vi "Tosca-Initialize Stimulus Generation.vi"(0 "Tosca":refnum<class "Parameters.lvclass">, 1 "StimCon in":T1, 11 "error in (no error)":errorcluster, 12 "SG Runtime":T7) -> (3 "StimCon out":T1, 4 "Tosca out":refnum<class "Parameters.lvclass">, 8 "AODO":T4[](array[typedef]), 15 "error out":errorcluster)   [LabVIEW 2020]
uses:
  Typedefs/Tosca-SG Runtime Params.ctl
  Typedefs/Tosca-AO Runtime.ctl
  Typedefs/Tosca-DO Runtime.ctl
  Imaging VIs/Tosca-Imaging Mode.ctl
  Classes/Parameters/Parameters.lvclass
  Typedefs/Tosca-State AODO.ctl
  epl-vi-lib/Signal Synthesis VIs/4th Generation/Classes/SignalManager/SignalManager.lvclass
  Typedefs/Tosca-SCL Element.ctl
  Typedefs/Tosca-Schedule Mode.ctl
  Typedefs/Tosca-Event Type.ctl
  Classes/Parameters/Parameters.lvclass/Parameters.ctl
  Classes/State/State.lvclass/State.ctl
  epl-vi-lib/Signal Synthesis VIs/4th Generation/Classes/SignalManager/SignalManager.lvclass/SignalManager.ctl
  Classes/State/Read Name.vi
  Classes/State/Read SigMan.vi
  epl-vi-lib/Signal Synthesis VIs/4th Generation/Classes/SignalManager/Read Interval (ms).vi
  Classes/Parameters/Read First state.vi
  Classes/Parameters/Read Flowchart.vi
  Classes/Parameters/Read DAQ.vi
  Classes/State/State.lvclass
  epl-vi-lib/PXI DAQ VIs/AODO/Typedefs/AODO-Action.ctl
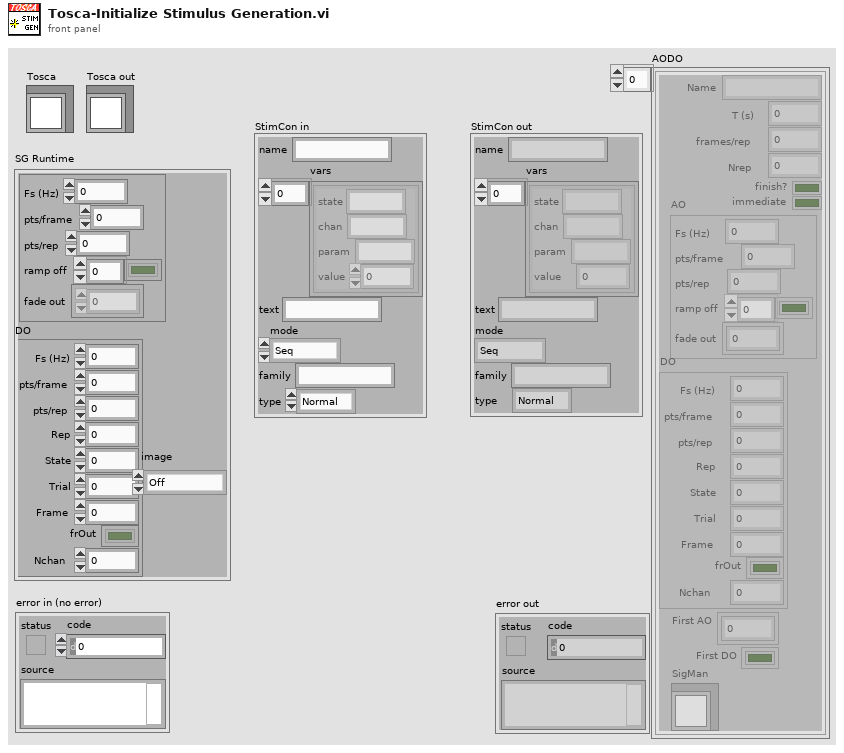
[diagram p1: front panel]
types:
  T1 = typedef "Tosca-SCL Element.ctl" = cluster{"name":string, "vars":cluster{"state":string, "chan":string, "param":string, "value":dbl}[], "text":string, "mode":T2, "family":string, "type":T3}
  T2 = typedef "Tosca-Schedule Mode.ctl" = enum16{"Seq", "CS+/CS-", "Adapt"}
  T3 = typedef "Tosca-Event Type.ctl" = enum16{"Normal", "CS+", "CS-"}
  T4 = typedef "Tosca-State AODO.ctl" = cluster{"Name":string, "T (s)":dbl, "First AO":dbl[][], "frames/rep":i32, "finish?":bool, "Nrep":i32, "AO":T5, "DO":T6, "immediate":bool, "First DO":bool[][], "SigMan":refnum<class "SignalManager.lvclass">}
  T5 = typedef "Tosca-AO Runtime.ctl" = cluster{"Fs (Hz)":dbl, "pts/frame":i32, "pts/rep":i32, "ramp off":bool[], "fade out":dbl[][]}
  T6 = typedef "Tosca-DO Runtime.ctl" = cluster{"Fs (Hz)":dbl, "pts/frame":i32, "pts/rep":i32, "Rep":i32, "State":i32, "Trial":i32, "Frame":i32, "frOut":bool[], "Nchan":i32}
  T7 = typedef "Tosca-SG Runtime Params.ctl" = cluster{"AO":T5, "DO":T6, "image":T8}
  T8 = typedef "Tosca-Imaging Mode.ctl" = enum16{"Off", "Widefield", "Two-photon"}
  T9 = typedef "Parameters.lvclass/DAQ.ctl" = cluster{"AO Fs (Hz)":dbl, "DO Fs (Hz)":dbl, "Poll Rate (Hz)":dbl, "Baseline (s)":dbl}
  T10 = typedef "AODO-Action.ctl" = enum16{"Configure", "Initialize", "Start", "Write", "Clean up", "Init & Start", "Config & Test", "Position", "Set AO Gains", "Zero"}
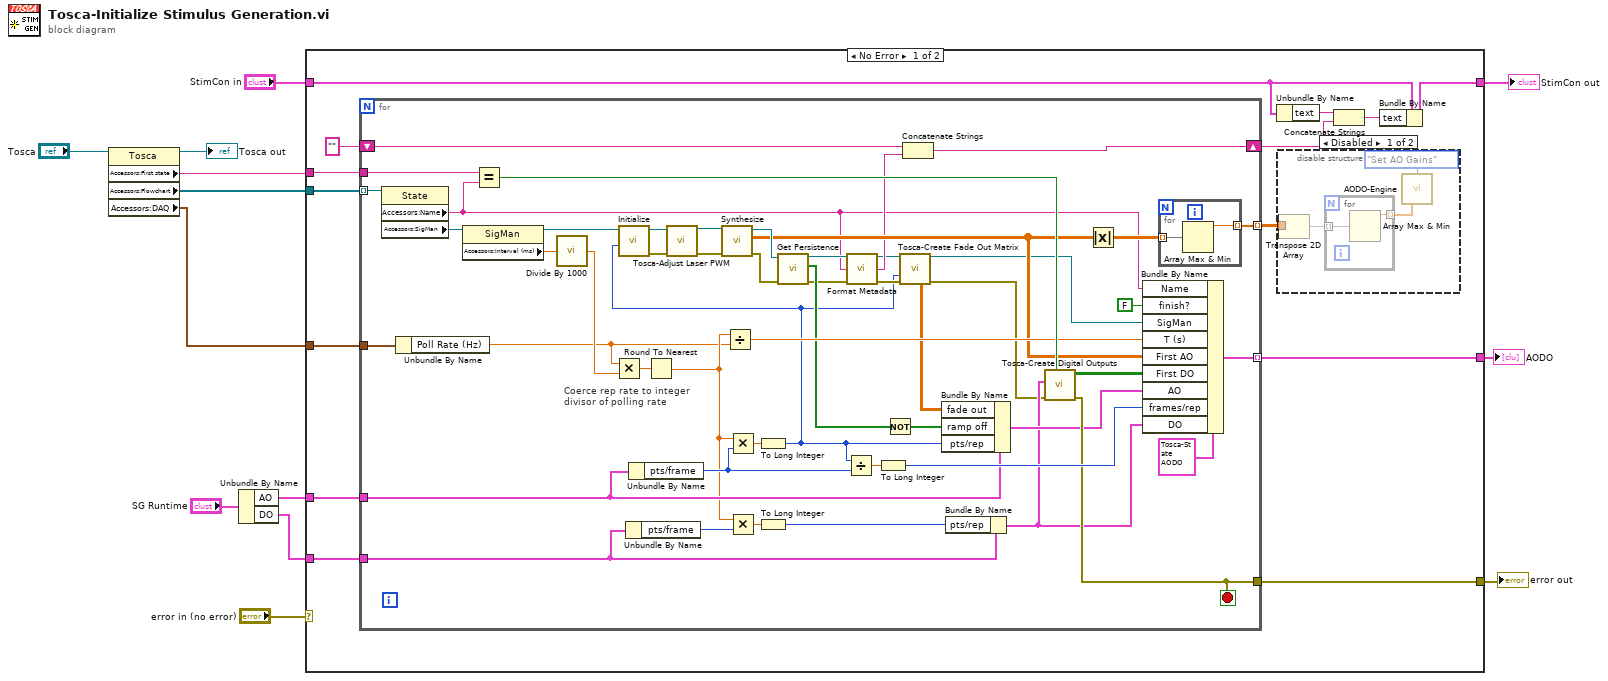
[diagram p0: block diagram]
diagram:
  n1 = property class="Tosca"(reference="Tosca") -> (reference out=→"Tosca out":refnum<class "Parameters.lvclass">, "Accessors:First state"=w7:string, "Accessors:Flowchart"=w8:refnum<class "State.lvclass">[], "Accessors:DAQ"=w4:T9)  [unwired: 1 in, 1 out]
  n2 = Unbundle By Name("SG Runtime") -> ("AO"=w11:T5, "DO"=w10:T6)
  n3 = case shown="No Error" "error in (no error)" {
    selector: "error in (no error)" -> [_ w88]
    tunnel: [w25 w88] -> w12
    tunnel: [w22 _] -> w3
    tunnel: w11 -> [w27 _]
    tunnel: w10 -> [w26 _]
    tunnel: w8 -> [w24 _]
    tunnel: w7 -> [w23 _]
    tunnel: w4 -> [w21 _]
    tunnel: [w18 w87] -> w2
    tunnel: "StimCon in" -> [w17 w87]
    frame No Error {
      n4 = for {
        tunnel: w27 -> [w73]
        tunnel: w26 -> [w65]
        tunnel: [w69] -> w25
        tunnel: w24 -> [w61] mode=indexing
        tunnel: w23 -> [w57]
        tunnel: [w55] -> w22 mode=indexing
        tunnel: w21 -> [w54]
        tunnel: [w49] -> w20 mode=indexing
        shift-right: [w36] -> w15
        shift-left: "" -> [w39]
        stop <- w69 stop-if-true
        # "Coerce rep rate to integer divisor of polling rate"
        n5 = property class="State"(reference=w61) -> ("Accessors:Name"=w34:string, "Accessors:SigMan"=w58:refnum<class "SignalManager.lvclass">)  [unwired: 1 in, 2 out]
        n6 = Unbundle By Name(w54) -> ("Poll Rate (Hz)"=w53:dbl)
        n7 = property class="SigMan"(reference=w58) -> (reference out=w56:refnum<class "SignalManager.lvclass">, "Accessors:Interval (ms)"=w60:dbl)  [unwired: 1 in, 1 out]
        n8 = Equal?(x=w57, y=w34) -> (x = y?=w70:bool)
        n9 = call "Divide By 1000.vi"("X"=w60) -> ("X/1000"=w59:dbl)
        n10 = Multiply(x=w53, y=w59) -> (x*y=w78:dbl)
        n11 = Unbundle By Name(w65) -> ("pts/frame"=w62:i32)
        n12 = Unbundle By Name(w73) -> ("pts/frame"=w66:i32)
        n13 = Round To Nearest(number=w78) -> (nearest integer value=w63:dbl)
        n14 = Divide(x=w63, y=w53) -> (x/y=w64:dbl)
        n15 = Multiply(x=w63, y=w66) -> (x*y=w77:dbl)
        n16 = Multiply(x=w63, y=w62) -> (x*y=w74:dbl)
        n17 = To Long Integer(number=w77) -> (32bit integer=w29:i32)
        n18 = call "Initialize.vi"("Npts"=w29, "SigMan in"=w56) -> ("error out"=w46:errorcluster, "SigMan out"=w48:refnum<class "SignalManager.lvclass">)  [unwired: 8 in]
        n19 = call "Tosca-Adjust Laser PWM.vi"("SigMan in"=w48, "error in (no error)"=w46) -> ("SigMan out"=w47:refnum<class "SignalManager.lvclass">, "error out"=w45:errorcluster)  [unwired: 12 in]
        n20 = call "Synthesize.vi"("error in (no error)"=w45, "SigMan in"=w47) -> ("error out"=w44:errorcluster, "Array"=w40:dbl[][], "SigMan out"=w43:refnum<class "SignalManager.lvclass">)  [unwired: 7 in]
        n21 = To Long Integer(number=w74) -> (32bit integer=w72:i32)
        n22 = call "Get Persistence.vi"("error in (no error)"=w44, "SigMan in"=w43) -> ("error out"=w38:errorcluster, "persist"=w42:bool[], "SigMan out"=w37:refnum<class "SignalManager.lvclass">)  [unwired: 7 in]
        n23 = Divide(x=w29, y=w66) -> (x/y=w76:dbl)
        n24 = call "Format Metadata.vi"("SigMan in"=w37, "Prefix"=w34, "error in (no error)"=w38) -> ("SigMan out"=w32:refnum<class "SignalManager.lvclass">, "String"=w35:string, "error out"=w33:errorcluster)  [unwired: 10 in]
        n25 = To Long Integer(number=w76) -> (32bit integer=w75:i32)
        n26 = Not(x=w42) -> (.not. x?=w41:bool[])
        n27 = call "Tosca-Create Fade Out Matrix.vi"("SignalManager in"=w32, "npts"=w29, "error in (no error)"=w33) -> ("SignalManager out"=w31:refnum<class "SignalManager.lvclass">, "fade out"=w28:dbl[][], "error out"=w30:errorcluster)  [unwired: 10 in]
        n28 = Concatenate Strings(w39, w35) -> (w36:string)
        n29 = Bundle By Name(cluster=w73, "fade out"=w28, "ramp off"=w41, "pts/rep"=w29) -> (w68:T5)
        n30 = Bundle By Name(cluster=w65, "pts/rep"=w72) -> (w67:T6)
        n31 = call "Tosca-Create Digital Outputs.vi"("Trial start? (F)"=w70, "error in (no error)"=w30, "DO"=w67) -> ("error out"=w69:errorcluster, "DO Array"=w71:bool[][])  [unwired: 7 in]
        n32 = Absolute Value(x=w40) -> (abs(x)=w50:dbl[][])
        n33 = Bundle By Name(cluster=T4 {"Name"="", "T (s)"=0.0, "First AO"=[], "frames/rep"=0, "finish?"=FALSE, "Nrep"=0, "AO"={"Fs (Hz)"=0.0, "pts/frame"=0, "pts/rep"=0, "ramp off"=[], "fade out"=[]}, "DO"={"Fs (Hz)"=0.0, "pts/frame"=0, "pts/rep"=0, "Rep"=0, "State"=0, "Trial"=0, "Frame"=0, "frOut"=[], "Nchan"=0}, "immediate"=FALSE, "First DO"=[], "SigMan"=refnum} ("AODO"), "Name"=w34, "finish?"=FALSE ("Continue?"), "SigMan"=w31, "T (s)"=w64, "First AO"=w40, "First DO"=w71, "AO"=w68, "frames/rep"=w75, "DO"=w67) -> (w55:T4)
        n34 = for {
          tunnel: w50 -> [w80] mode=indexing
          tunnel: [w79] -> w49 mode=indexing
          n35 = Array Max & Min(array=w80) -> (max value=w79:dbl)  [unwired: 3 out]
        }
      }
      n36 = Unbundle By Name(w17) -> ("text"=w16:string)
      n37 = disable-structure shown="Disabled" {
        disable-tunnel: w20 -> [w84 _]
        frame Disabled {
          n38 = Transpose 2D Array(2D array=w84) -> (transposed array=w82:dbl[][])
          n39 = for {
            tunnel: w82 -> [w86] mode=indexing
            tunnel: [w85] -> w81 mode=indexing
            n40 = Array Max & Min(array=w86) -> (max value=w85:dbl)  [unwired: 3 out]
          }
          n41 = call "AODO-Engine.vi"("Action"=AODO-Action."Set AO Gains", "Vmax"=w81) -> ()  [unwired: 12 in, 2 out]
        }
        frame Enabled {
        }
      }
      n42 = Concatenate Strings(w16, w15) -> (w14:string)
      n43 = Bundle By Name(cluster=w17, "text"=w14) -> (w18:T1)
    }
    frame Error {
    }
  }
  "error out" <- w12
  "AODO" <- w3
  "StimCon out" <- w2
